vi "Calculate number of image bytes to read.vi"(9 "# of total images":u32, 10 "Total Images Read":u32, 11 "# of bytes per image":u32) -> (1 "All Images Read?":bool, 2 "# of Images Read":u32, 3 "# of bytes to read":u64)   [LabVIEW 2013]
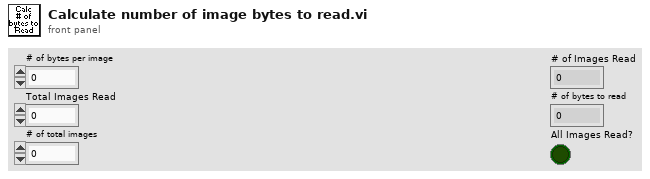
[diagram p1: front panel]
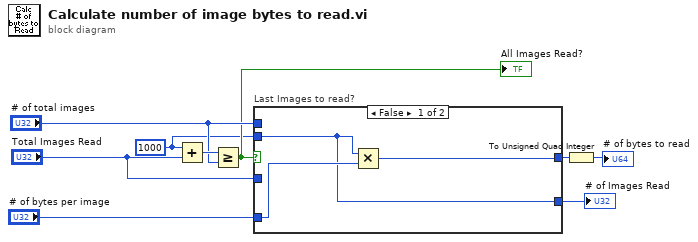
[diagram p0: block diagram]
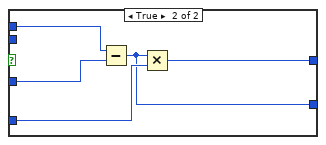
[diagram p2: hidden frame]
diagram:
  w3 = u32 1000 ("x")
  n1 = Add(x=w3, y="Total Images Read") -> (x+y=w9:u32)
  n2 = Greater Or Equal?(x=w9, y="# of total images") -> (x >= y?=w4:bool)
  "All Images Read?" <- w4
  n3 = case "Last Images to read?" shown="False" w4 {
    tunnel: "# of total images" -> [_ w17]
    tunnel: "Total Images Read" -> [_ w16]
    tunnel: "# of bytes per image" -> [w12 w15]
    tunnel: [w11 w14] -> w5
    tunnel: w3 -> [w10 _]
    tunnel: [w10 w13] -> w2
    frame False {
      n4 = Multiply(x=w10, y=w12) -> (x*y=w11:u32)
    }
    frame True {
      n5 = Subtract(x=w17, y=w16) -> (x-y=w13:u32)
      n6 = Multiply(x=w13, y=w15) -> (x*y=w14:u32)
    }
  }
  "# of Images Read" <- w2
  n7 = To Unsigned Quad Integer(1:w5) -> (0:→"# of bytes to read":u64)
